vi "BRig_comm_TCP_constants_byteRange_packet.vi"() -> (0 "output_end_byte":u8=62, 1 "output_end_char":string=">", 2 "output_start_byte":u8=60, 3 "output_start_char":string="<")   [LabVIEW 2014]
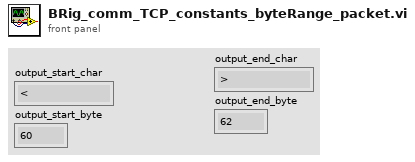
[diagram p1: front panel]
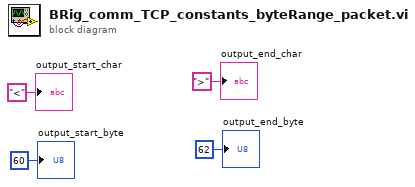
[diagram p0: block diagram]
diagram:
  "output_end_char" <- ">"
  "output_end_byte" <- u8 62
  "output_start_char" <- "<"
  "output_start_byte" <- u8 60
